vi "Serialize.vi"(8 "error in":errorcluster, 9 "OwningElement in":refnum<k20>, 10 "Document in":refnum<k20>, 11 "StringMeasure in":refnum<class "StringMeasure.lvclass">) -> (0 "error out":errorcluster, 1 "OwningElement out":refnum<k20>, 2 "Document out":refnum<k20>, 3 "StringMeasure out":refnum<class "StringMeasure.lvclass">)   [LabVIEW 2021, in "ProligentXMLGenerator.lvlib" / "StringMeasure.lvclass"]
uses:
  StringMeasure.lvclass
  StringMeasure.lvclass/StringMeasure.ctl
  Base/DOMSupport/DOMSupport.lvlib
  Measure/Measure.lvclass
  <vilib>/xml/NI_XML.lvlib
  <vilib>/xml/Close Reference(Node).vi
  MeasureLimit/MeasureLimit.lvclass
  Base/String_4000/String_4000.lvclass
  Base/Attribute/Attribute.lvclass
  C:/Projects/proligent-xml-generator-labview/src/ProligentXMLGenerator/Measure/Measure/Measure.lvclass
  Base/MeasureKind/MeasureKind.lvclass
  C:/Projects/proligent-xml-generator-labview/src/ProligentXMLGenerator/Base/Attribute/Attribute.lvclass
  C:/Projects/proligent-xml-generator-labview/src/ProligentXMLGenerator/Base/MeasureKind/MeasureKind.lvclass
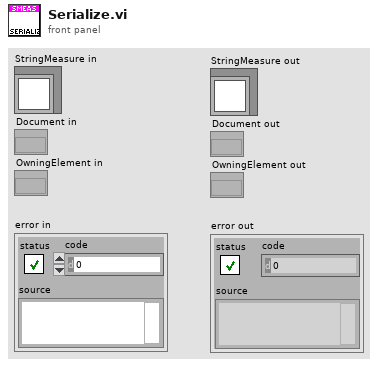
[diagram p1: front panel]
types:
  T1 = typedef "ProligentXMLGenerator.lvlib/StringMeasure.lvclass/Data.ctl" = cluster{"Value":refnum<class "String_4000.lvclass">}
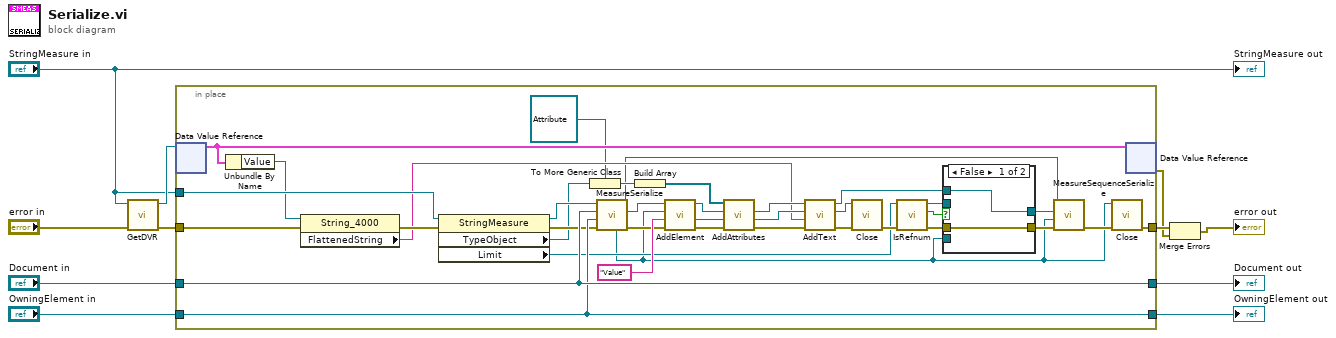
[diagram p0: block diagram]
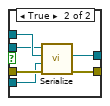
[diagram p2: hidden frame]
diagram:
  n1 = call "GetDVR.vi"("error in"="error in", "StringMeasure"="StringMeasure in") -> ("error out"=w4:errorcluster, "DVRReference"=w3:refnum<data-value>)  [unwired: 8 in]
  n2 = in-place "In Place Element Structure" {
    in-place-border: [w38] -> w5
    in-place-border: "Document in" -> [w47]
    in-place-border: w4 -> [w21]
    in-place-border: "OwningElement in" -> [w46]
    in-place-border: [w46] -> w7
    in-place-border: [w47] -> w6
    in-place-border: "StringMeasure in" -> [w41]
    n3 = in-place-dvr #1(w3) -> (w48:T1)  [unwired: 1 out]
    n4 = Unbundle By Name(w48) -> ("Value"=w22:refnum<class "String_4000.lvclass">)
    n5 = property on="Property Node" class="String_4000"(reference=w22, error in=w21) -> (error out=w23:errorcluster, "FlattenedString"=w20:string)  [unwired: 1 out]
    n6 = property on="Property Node" class="StringMeasure"(reference=w41, error in=w23) -> (reference out=w33:refnum<class "StringMeasure.lvclass">, error out=w42:errorcluster, "TypeObject"=w16:refnum<class "MeasureKind.lvclass">, "Limit"=w24:refnum<class "MeasureLimit.lvclass">)
    n7 = To More Generic Class(target class=refnum<class "Attribute.lvclass"> refnum ("ProligentResultProcessor:Attribute"), reference=w16) -> (generic class reference=w18:refnum<class "Attribute.lvclass">)
    n8 = call "MeasureSerialize.vi"("error in"=w42, "OwningElement in"=w46, "Document in"=w47, "Measure in"=w33) -> ("error out"=w43:errorcluster, "Document out"=w45:refnum<k20>, "Measure in"=w14:refnum<class "StringMeasure.lvclass">, "Element"=w12:refnum<k20>)  [unwired: 3 in, 1 out]
    n9 = Build Array(w18) -> (w19:refnum<class "Attribute.lvclass">[])
    n10 = call "AddElement.vi"("error in"=w43, "Name"="Value", "OwningElement in"=w12, "Document in"=w45) -> ("error out"=w37:errorcluster, "NewElement"=w39:refnum<k20>, "Document out"=w40:refnum<k20>)  [unwired: 4 in, 1 out]
    n11 = call "AddAttributes.vi"("error in"=w37, "OwningElement in"=w39, "Document in"=w40, "Attributes"=w19) -> ("error out"=w36:errorcluster, "OwningElement out"=w34:refnum<k20>, "Document out"=w35:refnum<k20>)  [unwired: 5 in]
    n12 = call "AddText.vi"("error in"=w36, "Text"=w20, "OwningElement in"=w34, "Document in"=w35) -> ("error out"=w32:errorcluster, "OwningElement out"=w31:refnum<k20>, "Document out"=w25:refnum<k20>)  [unwired: 5 in]
    n13 = call-poly <vilib>:"Close.vi"("error in (no error)"=w32, "node"=w31) -> ("error out"=w27:errorcluster)  [unwired: 7 in]
    n14 = call "IsRefnum.vi"("error in"=w27, "MeasureLimit in"=w24) -> ("error out"=w30:errorcluster, "IsRefnum"=w29:bool, "MeasureLimit out"=w28:refnum<class "MeasureLimit.lvclass">)  [unwired: 7 in]
    n15 = case shown="False" w29 {
      tunnel: w30 -> [w50 w54]
      tunnel: [w50 w56] -> w26
      tunnel: w28 -> [_ w53]
      tunnel: w25 -> [w49 w55]
      tunnel: w12 -> [_ w52]
      tunnel: [w49 w51] -> w13
      frame False {
      }
      frame True {
        n16 = call "Serialize.vi"("error in"=w54, "OwningElement in"=w52, "Document in"=w55, "MeasureLimit in"=w53) -> ("error out"=w56:errorcluster, "Document out"=w51:refnum<k20>)  [unwired: 4 in, 2 out]
      }
    }
    n17 = call "MeasureSequenceSerialize.vi"("error in"=w26, "OwningElement in"=w12, "Document in"=w13, "Measure in"=w14) -> ("error out"=w15:errorcluster)  [unwired: 4 in, 3 out]
    n18 = call-poly <vilib>:"Close.vi"("error in (no error)"=w15, "node"=w12) -> ("error out"=w38:errorcluster)  [unwired: 7 in]
    n19 = in-place-dvr #1(w48) -> (w2:errorcluster)  [unwired: 1 out]
  }
  "Document out" <- w6
  "OwningElement out" <- w7
  n20 = Merge Errors(w5, w2) -> (→"error out":errorcluster)
  "StringMeasure out" <- "StringMeasure in"
